vi "DAQ.vi"() -> ()   [LabVIEW 2014]
uses:
  <vilib>/Math Plots/2D Math Plots/2D Error Bar/2D Error Bar XCtrl/2D Error Bar.xctl
  <vilib>/Math Plots/2D Math Plots/2D Error Bar/2D Error Bar Datatype/2D Error Bar Datatype.lvclass
  <vilib>/Math Plots/2D Math Plots/2D Error Bar/2D Error Bar Datatype/Public/Plot Helper (Fixed).vi
  <vilib>/Utility/file.llb/Write To Spreadsheet File (DBL).vi
  <instrlib>/Zurich Instruments LabOne/Zurich Instruments LabOne.lvlib
panel:
  in  "Time constant (ms)":dbl=400.0
  in  "Comport (Monochromator):":refnum<visa-resource-name>="COM3"
  in  "FileName:":string="Measurement"
  in  "FilePath:":path=path "C:/Users/hebecked/Desktop/measurements/Results/New_Setup"
  in  "# (avg)":dbl=10.0
  in  "Intervall":dbl=4.0
  in  "Stop":dbl=700.0
  in  "Start":dbl=240.0
  out "Frequency (Hz)":dbl=330.0033881746923
  out "Monochromator error":bool
  out "Error Out":errorcluster
  out "Time left (sec):":dbl
  out "Time elapsed (sec):":dbl=513.707
  out "Path:":path=path "C:/Users/hebecked/Desktop/measurements/Results/New_Setup/Measurement_15h55m17s_20d03m2015.csv"
  in  "Start":bool
  out "Zero Measurement (No Signal!)":bool
  out "Signal:":cluster{"X":dbl, "Y":dbl}[](graph)=[{"X"=240.0, "Y"=0.0001124799275119779}, {"X"=244.0, "Y"=0.00010912916820628708}, {"X"=248.0, "Y"=0.00010695003730165524}, {"X"=252.0, "Y"=0.00010422874879095095}, {"X"=256.0, "Y"=0.0001054549589933801}, {"X"=260.0, "Y"=0.00010426769300193882}, {"X"=264.0, "Y"=0.0001086847718854195}, {"X"=268.0, "Y"=0.00012334638300290539}, {"X"=272.0, "Y"=0.0001435391589416127}, {"X"=276.0, "Y"=0.00017341189157166686}, {"X"=280.0, "Y"=0.00021228800994263462}, {"X"=284.0, "Y"=0.0002705065827922277}, {"X"=288.0, "Y"=0.0003870557900471551}, {"X"=292.0, "Y"=0.0004827077262718311}, {"X"=296.0, "Y"=0.0005448509377663002}, {"X"=300.0, "Y"=0.0005952325966221907}, {"X"=304.0, "Y"=0.00062350375235173}, {"X"=308.0, "Y"=0.0006559327078286819}, {"X"=312.0, "Y"=0.0006768712513392171}, {"X"=316.0, "Y"=0.000681013735603047}, {"X"=320.0, "Y"=0.0006842015488418314}, {"X"=324.0, "Y"=0.000676318924852958}, {"X"=328.0, "Y"=0.0006730004705153043}, {"X"=332.0, "Y"=0.0006937290902426208}, {"X"=336.0, "Y"=0.0006918971442294301}, {"X"=340.0, "Y"=0.0006847732251713362}, {"X"=344.0, "Y"=0.0006760619214817358}, {"X"=348.0, "Y"=0.000670501323843693}, {"X"=352.0, "Y"=0.000673216396152176}, {"X"=356.0, "Y"=0.0006774485740981105}, {"X"=360.0, "Y"=0.0006697903906472237}, {"X"=364.0, "Y"=0.000662059057938002}, {"X"=368.0, "Y"=0.0006655567270224821}, {"X"=372.0, "Y"=0.0006542323811675055}, {"X"=376.0, "Y"=0.0006563508066694601}, {"X"=380.0, "Y"=0.0006551932923552524}, {"X"=384.0, "Y"=0.0006502992356044546}, {"X"=388.0, "Y"=0.0006541992312091289}, {"X"=392.0, "Y"=0.0006450404199004142}, {"X"=396.0, "Y"=0.0006424534825636261}, {"X"=400.0, "Y"=0.0006404798484344894}, {"X"=404.0, "Y"=0.0006359342997841925}, {"X"=408.0, "Y"=0.0006385436387475234}, {"X"=412.0, "Y"=0.0006311654976092189}, {"X"=416.0, "Y"=0.0006241363441942785}, {"X"=420.0, "Y"=0.000616293060681249}, {"X"=424.0, "Y"=0.0006130769448085722}, {"X"=428.0, "Y"=0.0006072788677126594}, {"X"=432.0, "Y"=0.0006002595370205415}, {"X"=436.0, "Y"=0.000604254175550439}, {"X"=440.0, "Y"=0.0005971670501249255}, {"X"=444.0, "Y"=0.0005919112538931488}, {"X"=448.0, "Y"=0.0005941195253073914}, {"X"=452.0, "Y"=0.0005910579589660812}, {"X"=456.0, "Y"=0.0005928949075544557}, {"X"=460.0, "Y"=0.0005965086605133085}, {"X"=464.0, "Y"=0.0005926824080275991}, {"X"=468.0, "Y"=0.0005906592240422699}, {"X"=472.0, "Y"=0.0005955085034722927}, {"X"=476.0, "Y"=0.0005918713772908424}, {"X"=480.0, "Y"=0.0005916384972655447}, {"X"=484.0, "Y"=0.0005884875857267434}, {"X"=488.0, "Y"=0.0005834501883188729}, {"X"=492.0, "Y"=0.0005821518837124134}, {"X"=496.0, "Y"=0.0005847759712520804}, {"X"=500.0, "Y"=0.000584825170776149}, {"X"=504.0, "Y"=0.000581934668850303}, {"X"=508.0, "Y"=0.0005834582143282026}, {"X"=512.0, "Y"=0.0005842795728749178}, {"X"=516.0, "Y"=0.0005827358332372262}, {"X"=520.0, "Y"=0.0005843732943031112}, {"X"=524.0, "Y"=0.0005829746649759511}, {"X"=528.0, "Y"=0.0005819281093017439}, {"X"=532.0, "Y"=0.0005830255966573465}, {"X"=536.0, "Y"=0.0005823693373764331}, {"X"=540.0, "Y"=0.0005792226547527003}, {"X"=544.0, "Y"=0.0005757722880960276}, {"X"=548.0, "Y"=0.0005811540468580878}, {"X"=552.0, "Y"=0.0005804478134371961}, {"X"=556.0, "Y"=0.0005789816794623943}, {"X"=560.0, "Y"=0.0005793535815427208}, {"X"=564.0, "Y"=0.0005776447800366304}, {"X"=568.0, "Y"=0.0005791898163375316}, {"X"=572.0, "Y"=0.0005765502262541632}, {"X"=576.0, "Y"=0.0005743962786930696}, {"X"=580.0, "Y"=0.0005725800662436121}, {"X"=584.0, "Y"=0.0005748039741963212}, {"X"=588.0, "Y"=0.0005739875394208794}, {"X"=592.0, "Y"=0.0005728978956315848}, {"X"=596.0, "Y"=0.0005690361319835594}, {"X"=600.0, "Y"=0.0005702112754179914}, {"X"=604.0, "Y"=0.0005674957804657053}, {"X"=608.0, "Y"=0.0005669948538953433}, {"X"=612.0, "Y"=0.0005596890428600207}, {"X"=616.0, "Y"=0.0005581835048434785}, {"X"=620.0, "Y"=0.0005586790265475108}, {"X"=624.0, "Y"=0.0005572709315543228}, {"X"=628.0, "Y"=0.0005559676350746563}, {"X"=632.0, "Y"=0.0005538484696752859}, {"X"=636.0, "Y"=0.0005523170307747366}, {"X"=640.0, "Y"=0.0005496182115040158}, {"X"=644.0, "Y"=0.0005473316819791051}, {"X"=648.0, "Y"=0.0005453363428148616}, {"X"=652.0, "Y"=0.0005379231070060862}, {"X"=656.0, "Y"=0.0005363387364093823}, {"X"=660.0, "Y"=0.0005305977731438466}, {"X"=664.0, "Y"=0.0005289727034654906}, {"X"=668.0, "Y"=0.0005209055380840485}, {"X"=672.0, "Y"=0.0005205462615711712}, {"X"=676.0, "Y"=0.0005185233157566681}, {"X"=680.0, "Y"=0.0005144106616692233}, {"X"=684.0, "Y"=0.0005100831449910738}, {"X"=688.0, "Y"=0.000505716666510121}, {"X"=692.0, "Y"=0.000504437881015883}, {"X"=696.0, "Y"=0.0004971476770882843}, {"X"=700.0, "Y"=0.0004915778649578875}]
  out "Reference:":cluster{"X":dbl, "Y":dbl}[](graph)=[{"X"=240.0, "Y"=0.00027339419487120955}, {"X"=244.0, "Y"=0.00027156287640623945}, {"X"=248.0, "Y"=0.0002639574458568985}, {"X"=252.0, "Y"=0.0002531143715683025}, {"X"=256.0, "Y"=0.00024613742653185433}, {"X"=260.0, "Y"=0.00023685899984947234}, {"X"=264.0, "Y"=0.00023145871826484987}, {"X"=268.0, "Y"=0.0002304574751943674}, {"X"=272.0, "Y"=0.00023282840612288787}, {"X"=276.0, "Y"=0.00024290063228905824}, {"X"=280.0, "Y"=0.0002639817778834451}, {"X"=284.0, "Y"=0.00029490316866949336}, {"X"=288.0, "Y"=0.0003584082641364655}, {"X"=292.0, "Y"=0.00041425490318647827}, {"X"=296.0, "Y"=0.0004413722539305704}, {"X"=300.0, "Y"=0.000476415207299649}, {"X"=304.0, "Y"=0.0005029499002064922}, {"X"=308.0, "Y"=0.0005175104398873557}, {"X"=312.0, "Y"=0.0005259201048962571}, {"X"=316.0, "Y"=0.0005300989546073088}, {"X"=320.0, "Y"=0.0005443814900861256}, {"X"=324.0, "Y"=0.000539131275402185}, {"X"=328.0, "Y"=0.0005369362752596196}, {"X"=332.0, "Y"=0.0005349667311899773}, {"X"=336.0, "Y"=0.0005367341043363056}, {"X"=340.0, "Y"=0.0005365888229515568}, {"X"=344.0, "Y"=0.0005319169152469039}, {"X"=348.0, "Y"=0.0005367175543428894}, {"X"=352.0, "Y"=0.0005264345033744714}, {"X"=356.0, "Y"=0.000523955062124748}, {"X"=360.0, "Y"=0.0005255672871700865}, {"X"=364.0, "Y"=0.0005222503796038284}, {"X"=368.0, "Y"=0.000526572186350552}, {"X"=372.0, "Y"=0.0005174061504080259}, {"X"=376.0, "Y"=0.0005122007865471958}, {"X"=380.0, "Y"=0.0005123110087726367}, {"X"=384.0, "Y"=0.0005075233663995184}, {"X"=388.0, "Y"=0.0005100494788654713}, {"X"=392.0, "Y"=0.0005028812006166064}, {"X"=396.0, "Y"=0.000502763268724573}, {"X"=400.0, "Y"=0.0004960189757749436}, {"X"=404.0, "Y"=0.0004923721551170592}, {"X"=408.0, "Y"=0.0004946689002481598}, {"X"=412.0, "Y"=0.00048505829912491935}, {"X"=416.0, "Y"=0.00048163138181074616}, {"X"=420.0, "Y"=0.0004784451584899843}, {"X"=424.0, "Y"=0.0004831725383549942}, {"X"=428.0, "Y"=0.00048631584366838463}, {"X"=432.0, "Y"=0.0004890259617724656}, {"X"=436.0, "Y"=0.0004893297198012297}, {"X"=440.0, "Y"=0.00048462712539793163}, {"X"=444.0, "Y"=0.0004827647764432019}, {"X"=448.0, "Y"=0.0004702543520312838}, {"X"=452.0, "Y"=0.0004754781617881855}, {"X"=456.0, "Y"=0.00047669250749403906}, {"X"=460.0, "Y"=0.0004796860397123913}, {"X"=464.0, "Y"=0.0004803587525719171}, {"X"=468.0, "Y"=0.00048092930418125836}, {"X"=472.0, "Y"=0.000478494440240927}, {"X"=476.0, "Y"=0.00047905347559374143}, {"X"=480.0, "Y"=0.0004786749908812949}, {"X"=484.0, "Y"=0.0004772948377294158}, {"X"=488.0, "Y"=0.00047780447127344813}, {"X"=492.0, "Y"=0.0004773406077640608}, {"X"=496.0, "Y"=0.00047640549307784267}, {"X"=500.0, "Y"=0.0004769995379148509}, {"X"=504.0, "Y"=0.00047712179383849624}, {"X"=508.0, "Y"=0.0004769028147750848}, {"X"=512.0, "Y"=0.0004752652207538172}, {"X"=516.0, "Y"=0.000472601394469999}, {"X"=520.0, "Y"=0.0004762567787356515}, {"X"=524.0, "Y"=0.00047575754891499326}, {"X"=528.0, "Y"=0.00047270655562965495}, {"X"=532.0, "Y"=0.00047456887407592885}, {"X"=536.0, "Y"=0.00047586832394375523}, {"X"=540.0, "Y"=0.00047645330421502226}, {"X"=544.0, "Y"=0.0004738452769955132}, {"X"=548.0, "Y"=0.00047684526887240247}, {"X"=552.0, "Y"=0.0004782604143869107}, {"X"=556.0, "Y"=0.00047839137231198793}, {"X"=560.0, "Y"=0.0004805335413525478}, {"X"=564.0, "Y"=0.00048052239317865434}, {"X"=568.0, "Y"=0.00048004462332567043}, {"X"=572.0, "Y"=0.0004830723021826761}, {"X"=576.0, "Y"=0.00048098925433347445}, {"X"=580.0, "Y"=0.00048171985074294243}, {"X"=584.0, "Y"=0.0004819095127592272}, {"X"=588.0, "Y"=0.00048205776875935753}, {"X"=592.0, "Y"=0.0004841814644537626}, {"X"=596.0, "Y"=0.000478033286102336}, {"X"=600.0, "Y"=0.0004752652905179717}, {"X"=604.0, "Y"=0.00048055071133314836}, {"X"=608.0, "Y"=0.00048230419171126917}, {"X"=612.0, "Y"=0.0004789734769413004}, {"X"=616.0, "Y"=0.0004800266660899694}, {"X"=620.0, "Y"=0.0004812772186866619}, {"X"=624.0, "Y"=0.000479480311339967}, {"X"=628.0, "Y"=0.0004781125025591898}, {"X"=632.0, "Y"=0.00047919971142888887}, {"X"=636.0, "Y"=0.00047666134998792896}, {"X"=640.0, "Y"=0.0004758049511256013}, {"X"=644.0, "Y"=0.0004713053484591259}, {"X"=648.0, "Y"=0.000468238825902771}, {"X"=652.0, "Y"=0.00046981100003545026}, {"X"=656.0, "Y"=0.0004645608143796604}, {"X"=660.0, "Y"=0.00046465580527119653}, {"X"=664.0, "Y"=0.00046288526660319044}, {"X"=668.0, "Y"=0.0004596907609535929}, {"X"=672.0, "Y"=0.0004577042517276307}, {"X"=676.0, "Y"=0.0004528407487199883}, {"X"=680.0, "Y"=0.000449419698135344}, {"X"=684.0, "Y"=0.0004478156242068092}, {"X"=688.0, "Y"=0.0004431902752710935}, {"X"=692.0, "Y"=0.00044368442139343573}, {"X"=696.0, "Y"=0.0004377473949332918}, {"X"=700.0, "Y"=0.0004342396970892264}]
  out "Signal Phase:":refnum<class "2D Plot Datatype.lvclass">[](xcontrol)
  out "Reference Phase":refnum<class "2D Plot Datatype.lvclass">[](xcontrol)
  out "Result:":cluster{"X":dbl, "Y":dbl}[](graph)=[{"X"=240.0, "Y"=0.4114203213603892}, {"X"=244.0, "Y"=0.40185598875097095}, {"X"=248.0, "Y"=0.4051790884491168}, {"X"=252.0, "Y"=0.411785186851095}, {"X"=256.0, "Y"=0.4284393498350502}, {"X"=260.0, "Y"=0.44020996908794935}, {"X"=264.0, "Y"=0.46956439014345286}, {"X"=268.0, "Y"=0.5352240490306304}, {"X"=272.0, "Y"=0.6165019180084585}, {"X"=276.0, "Y"=0.7139211204905472}, {"X"=280.0, "Y"=0.8041767566106982}, {"X"=284.0, "Y"=0.9172725542850723}, {"X"=288.0, "Y"=1.0799298698642226}, {"X"=292.0, "Y"=1.1652432416823768}, {"X"=296.0, "Y"=1.234447641223971}, {"X"=300.0, "Y"=1.2493988174642996}, {"X"=304.0, "Y"=1.239693560125458}, {"X"=308.0, "Y"=1.267477247360374}, {"X"=312.0, "Y"=1.2870229623047718}, {"X"=316.0, "Y"=1.284691715922236}, {"X"=320.0, "Y"=1.2568420515796472}, {"X"=324.0, "Y"=1.2544605659325416}, {"X"=328.0, "Y"=1.2534084611621648}, {"X"=332.0, "Y"=1.2967705275793382}, {"X"=336.0, "Y"=1.2890873500296578}, {"X"=340.0, "Y"=1.2761600612638133}, {"X"=344.0, "Y"=1.2709915817734863}, {"X"=348.0, "Y"=1.249262891474822}, {"X"=352.0, "Y"=1.2788227060286232}, {"X"=356.0, "Y"=1.2929516728990345}, {"X"=360.0, "Y"=1.2744141558994386}, {"X"=364.0, "Y"=1.2677043115607316}, {"X"=368.0, "Y"=1.2639420468353502}, {"X"=372.0, "Y"=1.2644464714066088}, {"X"=376.0, "Y"=1.2814326410820178}, {"X"=380.0, "Y"=1.2788975468727957}, {"X"=384.0, "Y"=1.2813188094526944}, {"X"=388.0, "Y"=1.2826191542520486}, {"X"=392.0, "Y"=1.2826894684261405}, {"X"=396.0, "Y"=1.277844907392348}, {"X"=400.0, "Y"=1.2912406172240705}, {"X"=404.0, "Y"=1.2915724278376426}, {"X"=408.0, "Y"=1.29085058395057}, {"X"=412.0, "Y"=1.3012157481850894}, {"X"=416.0, "Y"=1.2958797282846672}, {"X"=420.0, "Y"=1.2881164115576487}, {"X"=424.0, "Y"=1.268857180699569}, {"X"=428.0, "Y"=1.2487334632814442}, {"X"=432.0, "Y"=1.2274594478479464}, {"X"=436.0, "Y"=1.2348609763492244}, {"X"=440.0, "Y"=1.2322196155128262}, {"X"=444.0, "Y"=1.2260862489887727}, {"X"=448.0, "Y"=1.2634003762879953}, {"X"=452.0, "Y"=1.243081189561307}, {"X"=456.0, "Y"=1.2437680438303715}, {"X"=460.0, "Y"=1.2435397554428753}, {"X"=464.0, "Y"=1.2338328485830294}, {"X"=468.0, "Y"=1.2281622660690585}, {"X"=472.0, "Y"=1.2445463382446993}, {"X"=476.0, "Y"=1.2355016870658833}, {"X"=480.0, "Y"=1.2359920792525034}, {"X"=484.0, "Y"=1.2329644890489349}, {"X"=488.0, "Y"=1.2211065894043582}, {"X"=492.0, "Y"=1.2195733491841503}, {"X"=496.0, "Y"=1.2274752910049476}, {"X"=500.0, "Y"=1.2260497637642285}, {"X"=504.0, "Y"=1.2196773997024448}, {"X"=508.0, "Y"=1.2234321045124696}, {"X"=512.0, "Y"=1.2293758250355311}, {"X"=516.0, "Y"=1.23303875116733}, {"X"=520.0, "Y"=1.227013074447955}, {"X"=524.0, "Y"=1.2253608299132108}, {"X"=528.0, "Y"=1.2310557202376928}, {"X"=532.0, "Y"=1.2285373704556635}, {"X"=536.0, "Y"=1.2238035357135173}, {"X"=540.0, "Y"=1.2156965848038248}, {"X"=544.0, "Y"=1.2151061032976795}, {"X"=548.0, "Y"=1.218747641624598}, {"X"=552.0, "Y"=1.2136647650031436}, {"X"=556.0, "Y"=1.2102678120307016}, {"X"=560.0, "Y"=1.2056464984983697}, {"X"=564.0, "Y"=1.2021183367033361}, {"X"=568.0, "Y"=1.2065332850204622}, {"X"=572.0, "Y"=1.1935071078369093}, {"X"=576.0, "Y"=1.1941977362655074}, {"X"=580.0, "Y"=1.188616299204898}, {"X"=584.0, "Y"=1.1927632864211712}, {"X"=588.0, "Y"=1.19070280912206}, {"X"=592.0, "Y"=1.1832297138386103}, {"X"=596.0, "Y"=1.190369266172276}, {"X"=600.0, "Y"=1.1997747085560195}, {"X"=604.0, "Y"=1.1809279792581164}, {"X"=608.0, "Y"=1.1755959488628582}, {"X"=612.0, "Y"=1.1685178194712693}, {"X"=616.0, "Y"=1.1628177021708632}, {"X"=620.0, "Y"=1.1608258293880347}, {"X"=624.0, "Y"=1.1622394462808292}, {"X"=628.0, "Y"=1.1628385204292542}, {"X"=632.0, "Y"=1.1557779699487039}, {"X"=636.0, "Y"=1.1587199817831328}, {"X"=640.0, "Y"=1.1551334432392855}, {"X"=644.0, "Y"=1.1613101437709923}, {"X"=648.0, "Y"=1.1646542589958138}, {"X"=652.0, "Y"=1.1449776760558958}, {"X"=656.0, "Y"=1.1545070522695047}, {"X"=660.0, "Y"=1.141915730148175}, {"X"=664.0, "Y"=1.142772824348617}, {"X"=668.0, "Y"=1.1331651238834346}, {"X"=672.0, "Y"=1.1372982872812296}, {"X"=676.0, "Y"=1.1450456197290988}, {"X"=680.0, "Y"=1.1446108477299255}, {"X"=684.0, "Y"=1.1390472270693002}, {"X"=688.0, "Y"=1.1410824982582954}, {"X"=692.0, "Y"=1.136929440595739}, {"X"=696.0, "Y"=1.1356953412916244}, {"X"=700.0, "Y"=1.1320426673401982}]
  # "Settings"
  # "Wavelength (nm):"
  # "Status"
  # "Data"
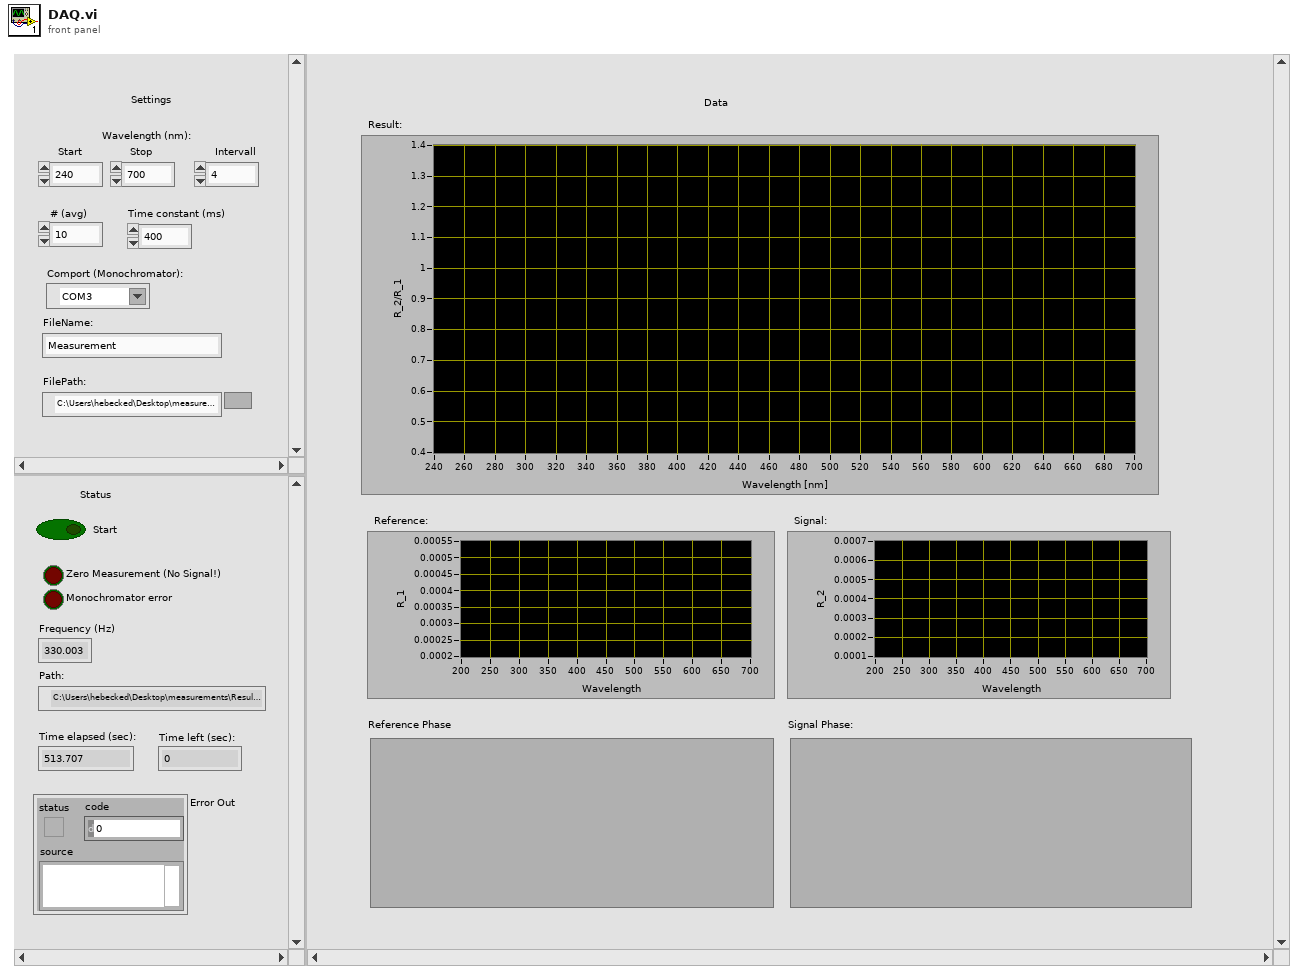
[diagram p1: front panel]
types:
  T1 = enum16{"open", "replace", "create", "open or create", "replace or create", "replace or create with confirmation"}
  T2 = typedef "Zurich Instruments LabOne.lvlib/ziTypeHandle.ctl" = cluster{"handleValid":bool, "Conn":u64, "Path Prefix":string, "EventBuffer":u8[], "Connected":bool, "Clockbase(s)":dbl}
  T3 = cluster{"error":bool, "code":i32, "source":string}
  T4 = cluster{"Frequency":dbl, "Error Frequency ":dbl, "R signal":dbl, "R signal error":dbl, "Theta signal":dbl, "Theta signal error":dbl, "R reference":dbl, "R reference error":dbl, "Theta reference":dbl, "Theta reference error":dbl, "R signal over R reference":dbl, "Theta signal error plus Theta reference error":dbl, "R signal over R reference error":dbl}
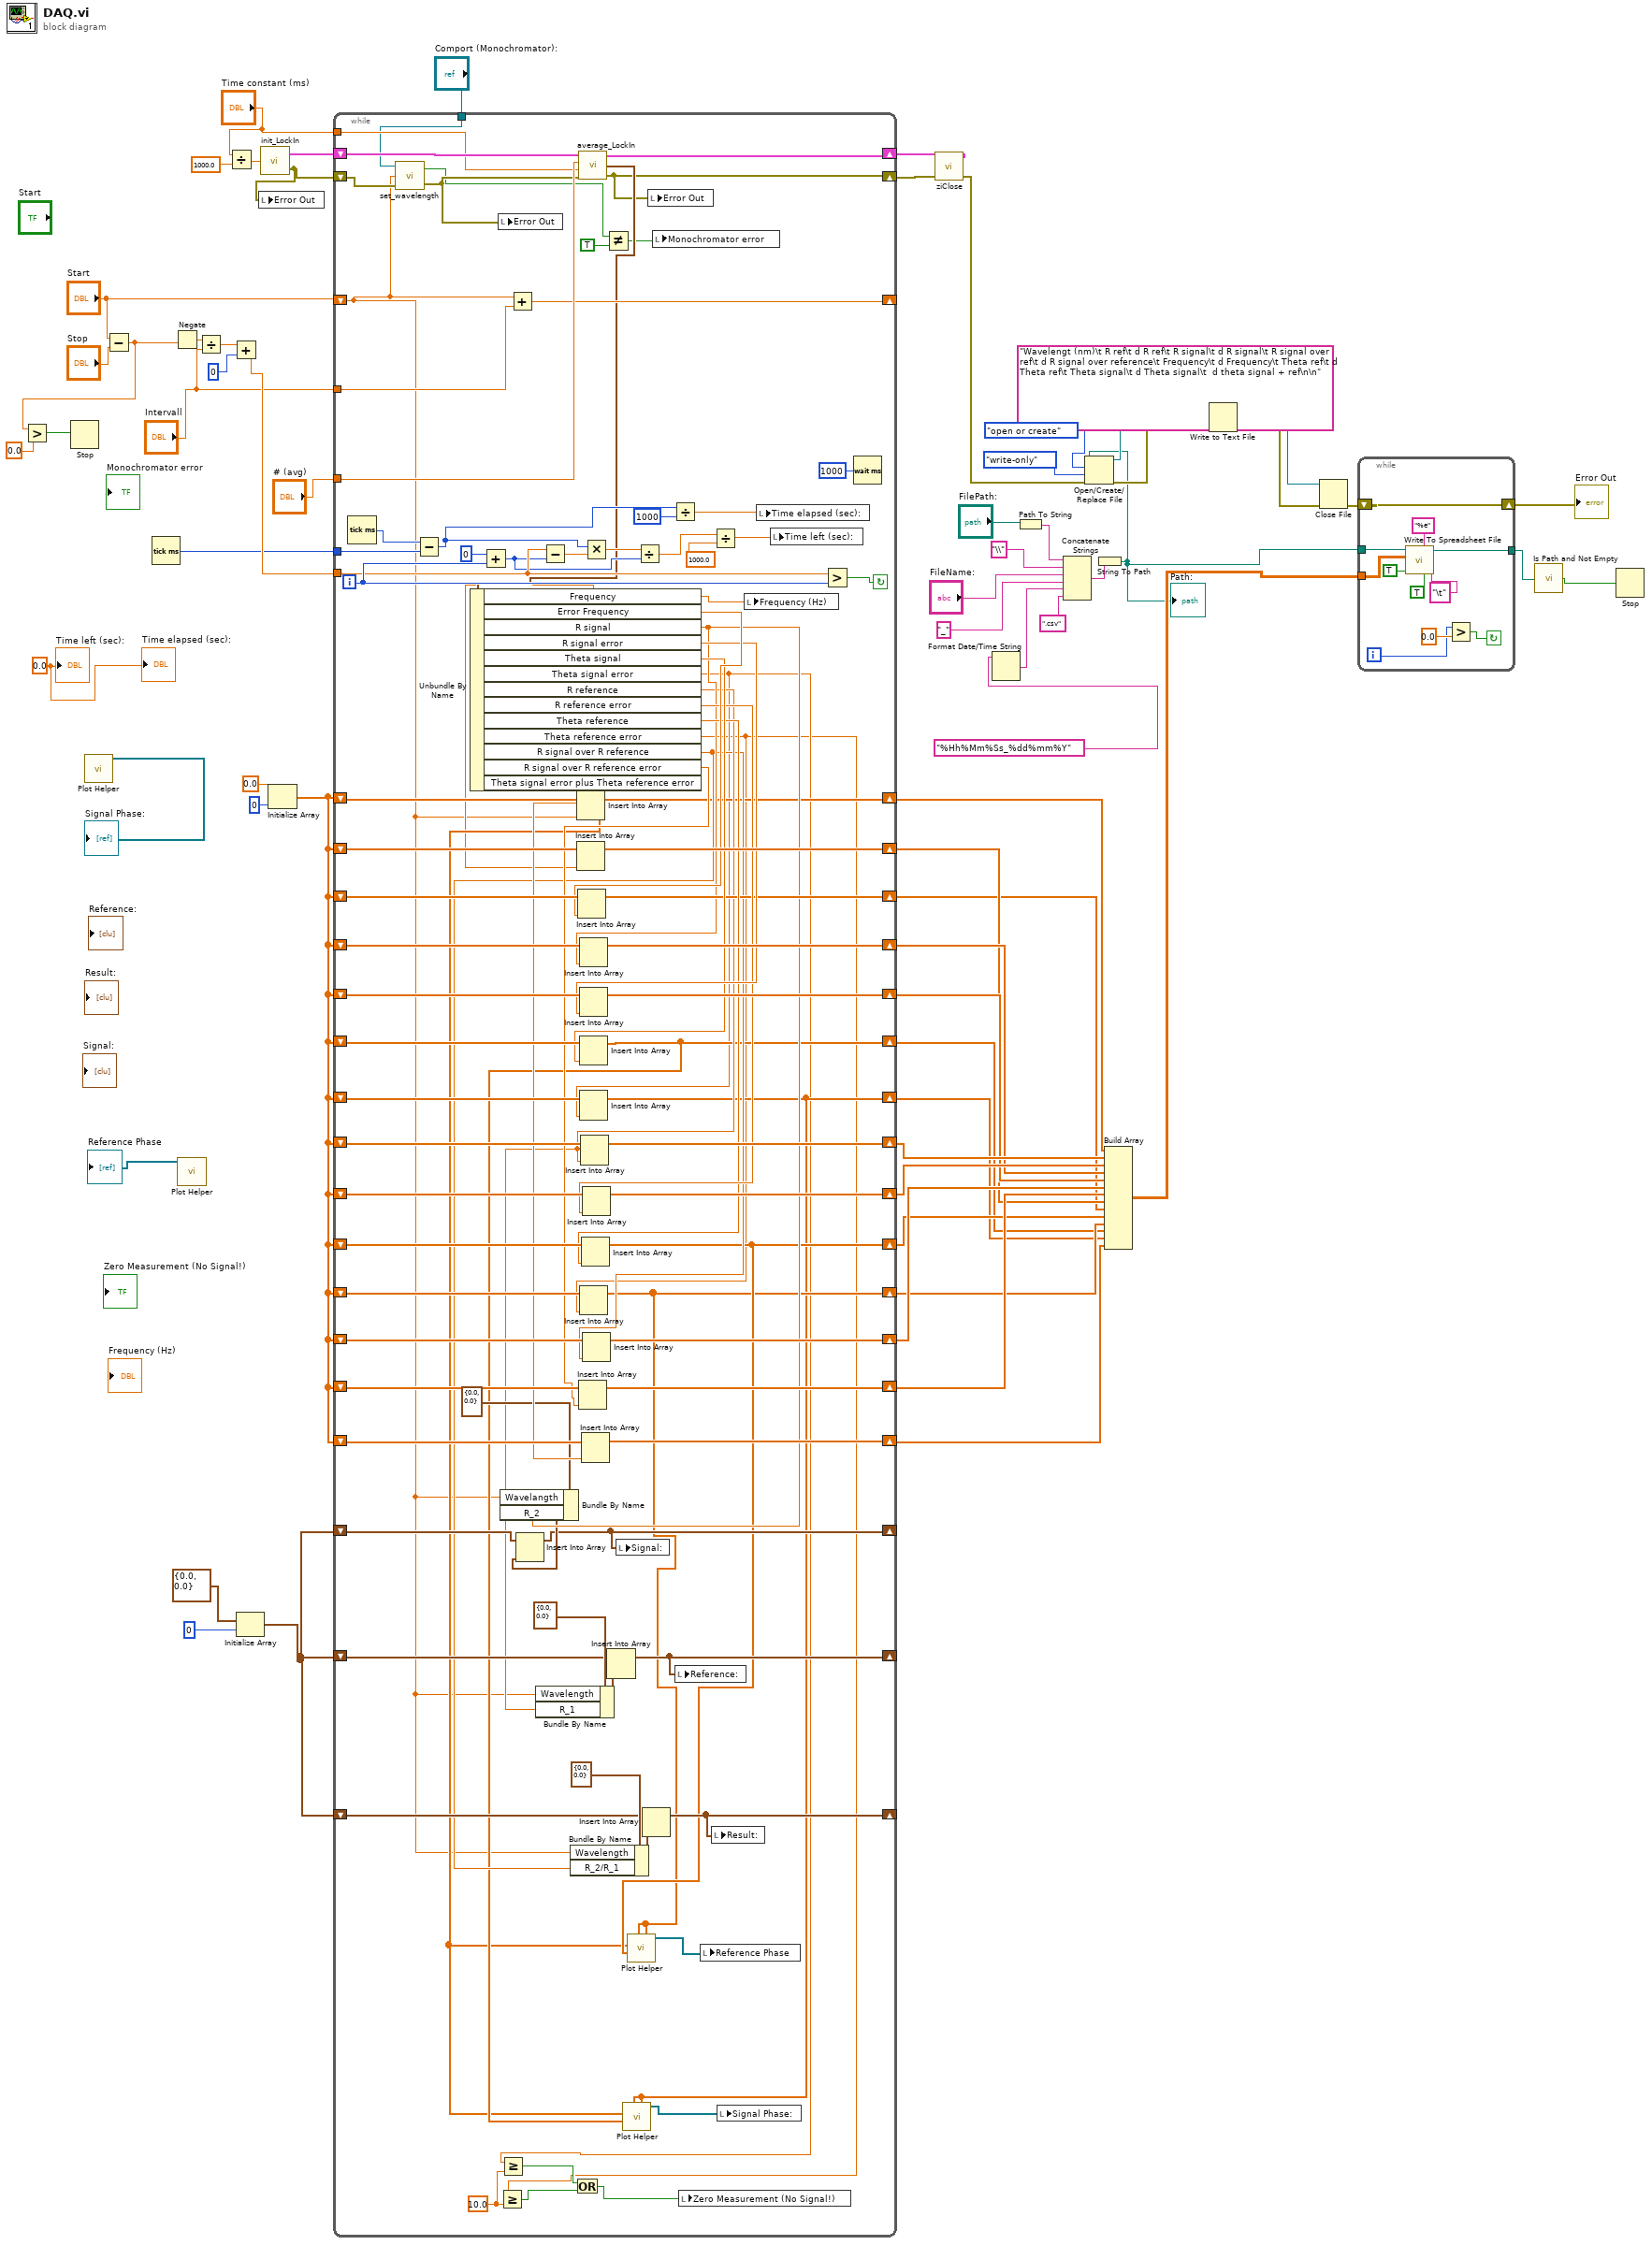
[diagram p0: block diagram]
diagram:
  w46 = 0.0 ("Time left (sec):")
  n1 = call-poly <vilib>:"Plot Helper.vi"() -> ("2D Plot Class Obj Array out"=→"Signal Phase:":refnum<class "2D Plot Datatype.lvclass">[])  [unwired: 6 in, 5 out]
  n2 = Subtract(x="Start", y="Stop") -> (x-y=w17:dbl)
  n3 = Greater?(x=w17, y=0.0 ("x")) -> (0:w18:bool)
  n4 = Stop(stop? (T)=w18) -> ()
  n5 = Tick Count (ms)() -> (millisecond timer value=w48:u32)
  n6 = Negate(x=w17) -> (-x=w19:dbl)
  n7 = call-poly <vilib>:"Plot Helper.vi"() -> ("2D Plot Class Obj Array out"=→"Reference Phase":refnum<class "2D Plot Datatype.lvclass">[])  [unwired: 6 in, 5 out]
  n8 = Divide(x=w19, y="Intervall") -> (x/y=w53:dbl)
  n9 = Divide(x="Time constant (ms)", y=1000.0) -> (x/y=w36:dbl)
  n10 = Add(x=w53, y=0) -> (x+y=w49:dbl)
  n11 = Initialize Array(cluster{"1.5":dbl, "1.5 2ho":dbl} {"1.5"=0.0, "1.5 2ho"=0.0} ("input cluster"), 0 ("dimension size")) -> (w39:cluster{"1.5":dbl, "1.5 2ho":dbl}[])
  n12 = call "init_LockIn.vi"("Timeconstant"=w36) -> ("Error Out"=w44:errorcluster, "HandleOut"=w45:T2)  [unwired: 2 in]
  n13 = local write "Error Out"(w44) -> ()
  n14 = Initialize Array(0.0 ("element"), 0 ("dimension size")) -> (w7:dbl[])
  n15 = while {
    shift-right: [w81] -> w63
    shift-left: w44 -> [w72]
    shift-right: [w139] -> w64
    shift-left: w45 -> [w140]
    tunnel: w49 -> [w151]
    tunnel: "# (avg)" -> [w138]
    tunnel: w48 -> [w154]
    tunnel: "Comport (Monochromator):" -> [w70]
    shift-right: [w137] -> _
    shift-left: "Start" -> [w71]
    tunnel: "Intervall" -> [w136]
    shift-right: [w82] -> w15
    shift-left: w7 -> [w114]
    shift-right: [w134] -> w8
    shift-left: w7 -> [w135]
    shift-right: [w106] -> w6
    shift-left: w7 -> [w133]
    shift-right: [w131] -> w12
    shift-left: w7 -> [w132]
    shift-right: [w83] -> w3
    shift-left: w7 -> [w115]
    shift-right: [w121] -> w1
    shift-left: w7 -> [w122]
    shift-right: [w116] -> w9
    shift-left: w7 -> [w123]
    shift-right: [w117] -> w10
    shift-left: w7 -> [w124]
    shift-right: [w86] -> w4
    shift-left: w7 -> [w125]
    shift-right: [w87] -> w5
    shift-left: w7 -> [w126]
    shift-right: [w118] -> w13
    shift-left: w7 -> [w127]
    shift-right: [w119] -> w14
    shift-left: w7 -> [w128]
    shift-right: [w84] -> w2
    shift-left: w7 -> [w129]
    shift-right: [w120] -> w11
    shift-left: w7 -> [w130]
    shift-right: [w100] -> _
    shift-left: w39 -> [w103]
    shift-right: [w95] -> _
    shift-left: w39 -> [w98]
    shift-right: [w90] -> _
    shift-left: w39 -> [w92]
    tunnel: "Time constant (ms)" -> [w89]
    i -> [w153]
    stop <- w156 continue-if-true
    w76 = 10.0 ("y")
    n16 = Tick Count (ms)() -> (millisecond timer value=w155:u32)
    n17 = call "set_wavelength.vi"("error in (no error)"=w72, "Wavelength"=w71, "Monochromator"=w70) -> ("error"=w69:T3, "Monochromator OK"=w68:bool)
    n18 = Subtract(x=w155, y=w154) -> (x-y=w143:u32)
    n19 = Add(x=0, y=w153) -> (x+y=w148:i32)
    n20 = local write "Error Out"(w69) -> ()
    n21 = Add(x=w71, y=w136) -> (x+y=w137:dbl)
    n22 = Subtract(x=w151, y=w148) -> (x-y=w150:dbl)
    n23 = Insert Into Array(array=w114, new element=w71) -> (w82:dbl[])  [unwired: 1 in]
    n24 = call "average_LockIn.vi"("error in"=w69, "Count(mSec)"=w89, "#AVG"=w138, "Handle In"=w140) -> ("Error Out"=w81:errorcluster, "output cluster"=w105:T4, "Handle Out"=w139:T2)
    n25 = Unbundle By Name(w105) -> ("Frequency"=w73:dbl, "Error Frequency"=w113:dbl, "R signal"=w104:dbl, "R signal error"=w112:dbl, "Theta signal"=w111:dbl, "Theta signal error"=w75:dbl, "R reference"=w97:dbl, "R reference error"=w110:dbl, "Theta reference"=w109:dbl, "Theta reference error"=w74:dbl, "R signal over R reference"=w91:dbl, "R signal over R reference error"=w108:dbl, "Theta signal error plus Theta reference error"=w107:dbl)
    n26 = Greater Or Equal?(x=w74, y=w76) -> (x >= y?=w78:bool)
    n27 = Greater Or Equal?(x=w75, y=w76) -> (x >= y?=w77:bool)
    n28 = Bundle By Name(cluster=cluster{"Wavelangth":dbl, "R_2":dbl} {"Wavelangth"=0.0, "R_2"=0.0} ("input cluster"), "Wavelangth"=w71, "R_2"=w104) -> (w102:cluster{"Wavelangth":dbl, "R_2":dbl})
    n29 = Insert Into Array(array=w103, new element=w102) -> (w100:cluster{"1.5":dbl, "1.5 2ho":dbl}[])  [unwired: 1 in]
    n30 = Bundle By Name(cluster=cluster{"Wavelength":dbl, "R_1":dbl} {"Wavelength"=0.0, "R_1"=0.0} ("input cluster"), "Wavelength"=w71, "R_1"=w97) -> (w96:cluster{"Wavelength":dbl, "R_1":dbl})
    n31 = Bundle By Name(cluster=cluster{"Wavelength":dbl, "R_2/R_1":dbl} {"Wavelength"=0.0, "R_2/R_1"=0.0} ("input cluster"), "Wavelength"=w71, "R_2/R_1"=w91) -> (w93:cluster{"Wavelength":dbl, "R_2/R_1":dbl})
    n32 = Or(x=w77, y=w78) -> (x .or. y?=w79:bool)
    n33 = Insert Into Array(array=w135, new element=w73) -> (w134:dbl[])  [unwired: 1 in]
    n34 = Insert Into Array(array=w133, new element=w113) -> (w106:dbl[])  [unwired: 1 in]
    n35 = Insert Into Array(array=w123, new element=w108) -> (w116:dbl[])  [unwired: 1 in]
    n36 = Insert Into Array(array=w132, new element=w104) -> (w131:dbl[])  [unwired: 1 in]
    n37 = Insert Into Array(array=w130, new element=w112) -> (w120:dbl[])  [unwired: 1 in]
    n38 = Insert Into Array(array=w115, new element=w111) -> (w83:dbl[])  [unwired: 1 in]
    n39 = Insert Into Array(array=w129, new element=w75) -> (w84:dbl[])  [unwired: 1 in]
    n40 = Insert Into Array(array=w125, new element=w74) -> (w86:dbl[])  [unwired: 1 in]
    n41 = Insert Into Array(array=w128, new element=w97) -> (w119:dbl[])  [unwired: 1 in]
    n42 = Insert Into Array(array=w126, new element=w109) -> (w87:dbl[])  [unwired: 1 in]
    n43 = Insert Into Array(array=w122, new element=w107) -> (w121:dbl[])  [unwired: 1 in]
    n44 = Multiply(x=w143, y=w150) -> (x*y=w149:dbl)
    n45 = Insert Into Array(array=w127, new element=w110) -> (w118:dbl[])  [unwired: 1 in]
    n46 = Insert Into Array(array=w124, new element=w91) -> (w117:dbl[])  [unwired: 1 in]
    n47 = Not Equal?(x=w68, y=TRUE) -> (x != y?=w80:bool)
    n48 = Insert Into Array(array=w98, new element=w96) -> (w95:cluster{"1.5":dbl, "1.5 2ho":dbl}[])  [unwired: 1 in]
    n49 = local write "Signal:"(w100) -> ()
    n50 = call-poly <vilib>:"Plot Helper.vi"("error b vector"=w84, "error a vector"=w84, "y vector"=w83, "x vector"=w82) -> ("2D Plot Class Obj Array out"=w85:refnum<class "2D Plot Datatype.lvclass">[])  [unwired: 2 in, 5 out]
    n51 = call-poly <vilib>:"Plot Helper.vi"("error b vector"=w86, "error a vector"=w86, "y vector"=w87, "x vector"=w82) -> ("2D Plot Class Obj Array out"=w88:refnum<class "2D Plot Datatype.lvclass">[])  [unwired: 2 in, 5 out]
    n52 = Divide(x=w149, y=w148) -> (x/y=w147:dbl)
    n53 = Insert Into Array(array=w92, new element=w93) -> (w90:cluster{"1.5":dbl, "1.5 2ho":dbl}[])  [unwired: 1 in]
    n54 = local write "Error Out"(w81) -> ()
    n55 = local write "Monochromator error"(w80) -> ()
    n56 = Divide(x=w143, y=u32 1000) -> (x/y=w144:dbl)
    n57 = local write "Reference:"(w95) -> ()
    n58 = local write "Zero Measurement (No Signal!)"(w79) -> ()
    n59 = local write "Reference Phase"(w88) -> ()
    n60 = Divide(x=w147, y=1000.0) -> (x/y=w145:dbl)
    n61 = local write "Result:"(w90) -> ()
    n62 = local write "Signal Phase:"(w85) -> ()
    n63 = local write "Frequency (Hz)"(w73) -> ()
    n64 = local write "Time elapsed (sec):"(w144) -> ()
    n65 = local write "Time left (sec):"(w145) -> ()
    n66 = Greater?(x=w151, y=w153) -> (0:w156:bool)
    n67 = Wait (ms)(milliseconds to wait=u32 1000) -> ()  [unwired: 1 out]
  }
  n68 = call <instrlib>:"ziClose.vi"("Error In"=w63, "Handle In"=w64) -> ("Error Out"=w33:errorcluster)  [unwired: 2 in, 1 out]
  n69 = Format Date/Time String(time format string (%c)="%Hh%Mm%Ss_%dd%mm%Y") -> (date/time string=w55:string)  [unwired: 2 in]
  n70 = Path To String(path="FilePath:") -> (string=w61:string)
  n71 = Concatenate Strings(w61, "\\", "FileName:", "_", w55, ".csv") -> (w60:string)
  n72 = String To Path(string=w60) -> (path=w22:path)
  "Path:" <- w22
  n73 = Open/Create/Replace File(file path (use dialog)=w22, error in=w33, operation (0:open)=T1."open or create", access (0:read/write)=enum16{"read/write", "read-only", "write-only"}."write-only") -> (refnum out=w30:refnum<file>, error out=w28:errorcluster)  [unwired: 2 in, 1 out]
  n74 = Build Array(w15, w14, w13, w12, w11, w10, w9, w8, w6, w5, w4, w3, w2, w1) -> (w23:dbl[][])
  n75 = Write to Text File(file (use dialog)=w30, text="Wavelengt (nm)\t R ref\t d R ref\t R signal\t d R signal\t R signal over ref\t d R signal over reference\t Frequency\t d Frequency\t Theta ref\t d Theta ref\t Theta signal\t d Theta signal\t  d theta signal + ref\n\n", error in=w28) -> (refnum out=w29:refnum<file>, error out=w27:errorcluster)  [unwired: 1 in, 1 out]
  n76 = Close File(refnum=w29, error in=w27) -> (error out=w25:errorcluster)  [unwired: 1 out]
  n77 = while {
    shift-right: [w164] -> w24
    shift-left: w25 -> [w164]
    tunnel: w23 -> [w159]
    tunnel: w22 -> [w158]
    tunnel: [w157] -> w21
    i -> [w165]
    stop <- w167 continue-if-true
    n78 = call-poly <vilib>:"Write To Spreadsheet File.vi"("delimiter (\\t)"="\t" ("delimiter (\\t)"), "transpose? (no:F)"=TRUE, "format (%.3f)"="%e", "append to file? (new file:F)"=TRUE, "2D data"=w159, "file path (dialog if empty)"=w158) -> ("new file path (Not A Path if cancelled)"=w157:path)  [unwired: 2 in]
    n79 = Greater?(x=w165, y=0.0) -> (0:w167:bool)
  }
  "Error Out" <- w24
  n80 = call <vilib>:"Is Path and Not Empty.vi"("path"=w21) -> ("Is Path and Not Empty?"=w20:bool)  [unwired: 4 in]
  n81 = Stop(stop? (T)=w20) -> ()
  "Time elapsed (sec):" <- w46
  "Time left (sec):" <- w46
